vi "Read Version.vi"(8 "error in (no error)":errorcluster, 11 "ByteRESTBase in":refnum<class "RESTBase.lvclass">) -> (0 "error out":errorcluster, 2 "Version":string, 3 "ByteRESTBase out":refnum<class "RESTBase.lvclass">)   [LabVIEW 2019, in "ByteREST.lvlib" / "RESTBase.lvclass"]
uses:
  RESTBase.lvclass
  RESTBase.lvclass/RESTBase.ctl
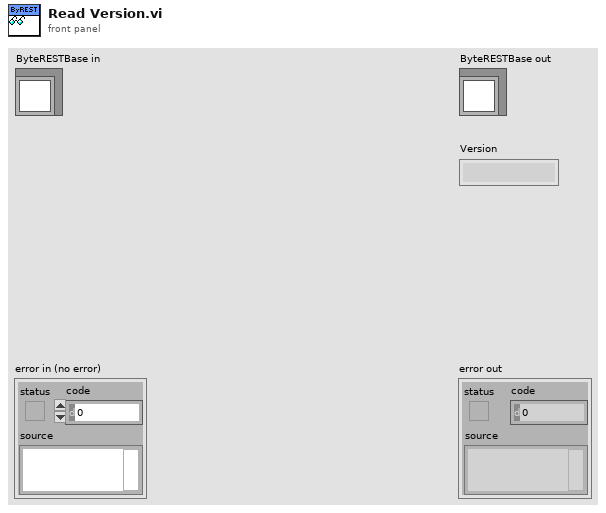
[diagram p1: front panel]
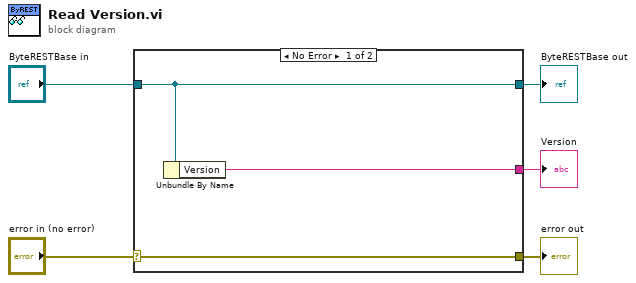
[diagram p0: block diagram]
diagram:
  n1 = case shown="No Error" "error in (no error)" {
    selector: "error in (no error)" -> [w8 w9]
    tunnel: [w8 w9] -> w4
    tunnel: [w7 w10] -> w2
    tunnel: "ByteRESTBase in" -> [w7 w10]
    tunnel: [w6 _] -> w1
    frame No Error {
      n2 = Unbundle By Name(w7) -> ("Version"=w6:string)
    }
    frame Error {
    }
  }
  "error out" <- w4
  "ByteRESTBase out" <- w2
  "Version" <- w1
